vi "查询启动项.vi"(8 "error in (no error)":errorcluster caption="错误输入（无错误）") -> (0 "error out":errorcluster caption="错误输出", 2 "values":string[](array[string]) caption="值", 3 "包含启动项":bool)   [LabVIEW 2016, in "wxpusher.lvlib"]
uses:
  wxpusher.lvlib
  <vilib>/registry/registry.llb/Registry RtKey.ctl
panel:
  out "value info":T1 caption="值信息"
  out "String/Binary data":string[](array[string]) caption="字符串/二进制数据"
  out "class":string caption="类"
  out "subkey info":T2 caption="子项信息"
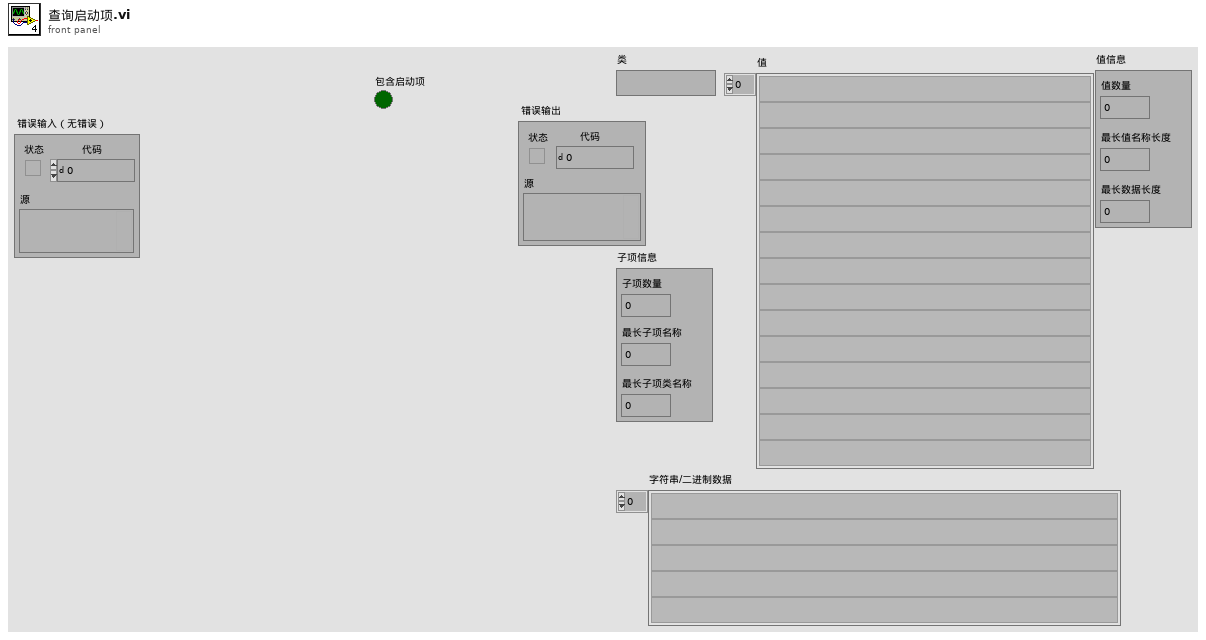
[diagram p1: front panel]
types:
  T1 = cluster{"numValues":i32, "maxValueNameLen":i32, "maxValueDataLen":i32}
  T2 = cluster{"numSubKeys":i32, "maxSubKeyLen":i32, "maxSubKeyClassLen":i32}
  T3 = typedef "Registry RtKey.ctl" = enum32{"HKEY_CLASSES_ROOT", "HKEY_CURRENT_USER", "HKEY_LOCAL_MACHINE", "HKEY_USERS", "HKEY_PERFORMANCE_DATA", "HKEY_CURRENT_CONFIG", "HKEY_DYN_DATA"}
  T4 = typedef "Registry refnum.ctl" = refnum<k1>
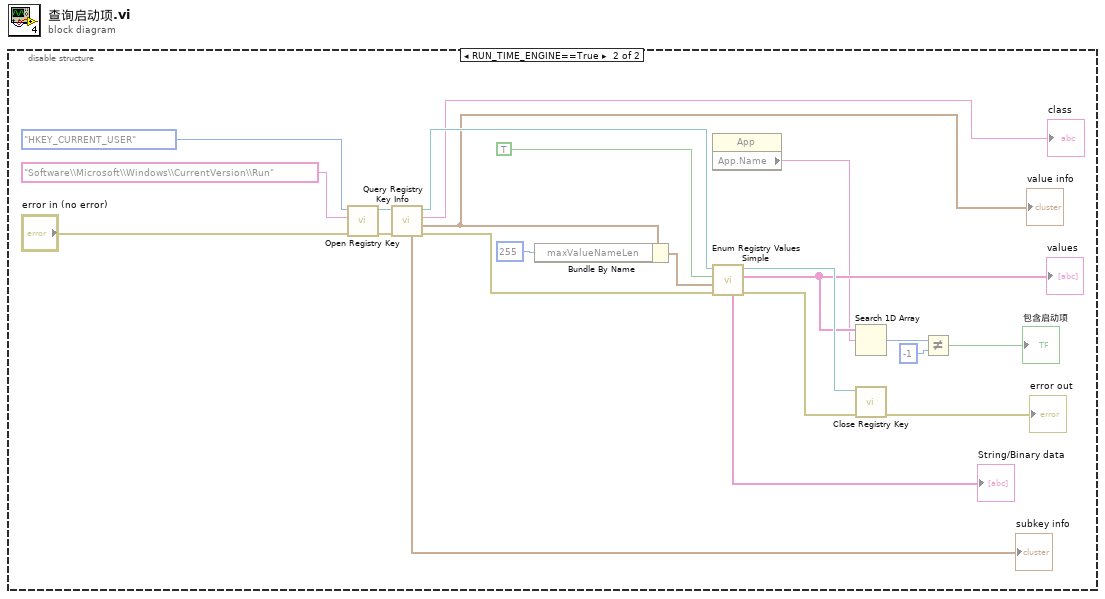
[diagram p0: block diagram]
diagram:
  n1 = disable-structure shown="RUN_TIME_ENGINE==True" {
    frame condition #0 (active) {
    }
    frame condition #1 {
      n2 = call <vilib>:"Open Registry Key.vi"("error in (no error)"="error in (no error)", "subkey"="Software\\Microsoft\\Windows\\CurrentVersion\\Run", "root key (HKEY_LOCAL_MACHINE)"=Registry_RtKey."HKEY_CURRENT_USER") -> ("error out"=w18:errorcluster, "refnum out"=w19:T4)  [unwired: 7 in]
      n3 = call <vilib>:"Query Registry Key Info.vi"("error in (no error)"=w18, "refnum"=w19) -> ("error out"=w16:errorcluster, "value info"=w3:T1, "class"=→"class":string, "refnum out"=w17:T4, "subkey info"=→"subkey info":T2)  [unwired: 5 in]
      "value info" <- w3
      n4 = Bundle By Name(cluster=w3, "maxValueNameLen"=255 ("numValues")) -> (w2:T1)
      n5 = property class="App"() -> ("App.Name"=w8:string)  [unwired: 2 in, 2 out]
      n6 = call <vilib>:"Enum Registry Values Simple.vi"("error in (no error)"=w16, "value info"=w2, "retrieve data? (F)"=TRUE, "refnum"=w17) -> ("error out"=w14:errorcluster, "values"=w13:string[], "refnum out"=w15:T4, "String/Binary data"=→"String/Binary data":string[])  [unwired: 2 in, 2 out]
      "values" <- w13
      n7 = Search 1D Array(1D array=w13, element=w8) -> (index of element=w12:i32)  [unwired: 1 in]
      n8 = call <vilib>:"Close Registry Key.vi"("error in (no error)"=w14, "refnum"=w15) -> ("error out"=→"error out":errorcluster)  [unwired: 5 in]
      n9 = Not Equal?(x=w12, y=-1) -> (x != y?=→"包含启动项":bool)
    }
  }
